vi "AI Ch to KH Ch.vi"(8 "error in (no error)":errorcluster, 11 "Number of AI":i32) -> (0 "error out":errorcluster, 3 "KH Ch []":string[](array[string]))   [LabVIEW 2016, in "Control Experiment UI.lvclass"]
uses:
  Control Experiment UI.lvclass
  Control Experiment SM/Control Experiment SM.lvclass
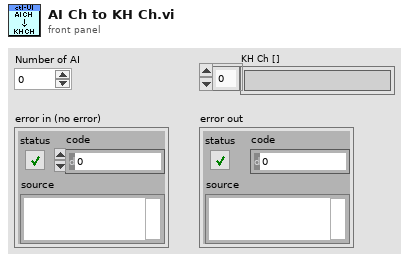
[diagram p1: front panel]
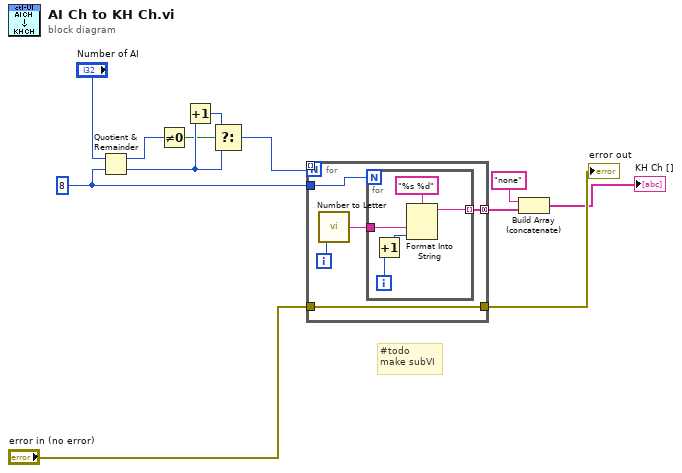
[diagram p0: block diagram]
diagram:
  w5 = 8 ("y")
  # "#todo\nmake subVI"
  n1 = Quotient & Remainder(x="Number of AI", y=w5) -> (x-y*floor(x/y)=w6:i32, floor(x/y)=w9:i32)
  n2 = Not Equal To 0?(x=w6) -> (x != 0?=w7:bool)
  n3 = Increment(x=w9) -> (x+1=w8:i32)
  n4 = Select(t=w8, s=w7, f=w9) -> (s? t:f=w10:i32)
  n5 = for {
    N: w10 -> [w14]
    tunnel: [w16] -> w2 mode=concatenating
    tunnel: w5 -> [w15]
    tunnel: [w14] -> _ mode=indexing
    tunnel: [w13] -> w12
    tunnel: "error in (no error)" -> [w13]
    i -> [w18]
    n6 = call "Number to Letter.vi"("Number"=w18) -> ("Letter"=w17:string)
    n7 = for {
      N: w15 -> [_]
      tunnel: w17 -> [w22]
      tunnel: [w20] -> w16 mode=indexing
      i -> [w21]
      n8 = Increment(x=w21) -> (x+1=w19:i32)
      n9 = Format Into String(format string="%s %d", w22, w19) -> (resulting string=w20:string)  [unwired: 2 in, 1 out]
    }
  }
  "error out" <- w12
  n10 = Build Array (concatenate)("none", w2) -> (→"KH Ch []":string[])
